vi "OAT Tachless Remove Control Point.vi"(10 "Pop Pos":cluster{i32, i32}, 11 "Tracks Ref":refnum<vi>) -> ()   [LabVIEW 2017, in "SoundVib_Tachless.lvlib"]
uses:
  <vilib>/addons/Sound and Vibration/Order Analysis/Tachless/SoundVib_Tachless.lvlib
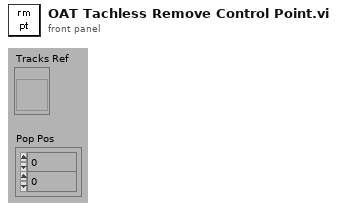
[diagram p1: front panel]
types:
  T1 = cluster{"Name":string, "Color":u32, "Style":u8, "Point Style":u8, "Name Visible":bool, "Allow Drag":bool, "Lock Style":u32, "Plot":u32, "Index":i32, "Position":cluster{"X":dbl, "Y":dbl}}[]
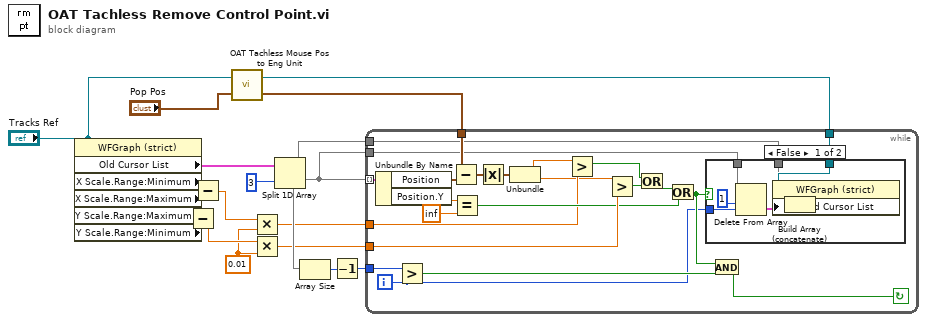
[diagram p0: block diagram]
diagram:
  w2 = 0.01 ("y")
  n1 = property on="Property Node" class="WFGraph (strict)"(reference="Tracks Ref") -> ("Old Cursor List"=w17:T1, "X Scale.Range:Minimum"=w11:dbl, "X Scale.Range:Maximum"=w12:dbl, "Y Scale.Range:Maximum"=w7:dbl, "Y Scale.Range:Minimum"=w6:dbl)  [unwired: 1 in, 2 out]
  n2 = Subtract(x=w7, y=w6) -> (x-y=w5:dbl)
  n3 = Subtract(x=w12, y=w11) -> (x-y=w3:dbl)
  n4 = call <vilib>:"OAT Tachless Mouse Pos to Eng Unit.vi"("Pop Pos"="Pop Pos", "Tracks ref"="Tracks Ref") -> ("Control Point"=w13:cluster{dbl, dbl})  [unwired: 1 in]
  n5 = Multiply(x=w3, y=w2) -> (x*y=w1:dbl)
  n6 = Multiply(x=w5, y=w2) -> (x*y=w4:dbl)
  n7 = Split 1D Array(array=w17, index=3 ("Array Index")) -> (first subarray=w9:T1, second subarray=w8:T1)
  n8 = Array Size(array=w8) -> (size(s)=w15:i32)
  n9 = Decrement(x=w15) -> (x-1=w14:i32)
  n10 = while {
    tunnel: w1 -> [w22]
    tunnel: w8 -> [w25]
    tunnel: w9 -> [w26]
    tunnel: "Tracks Ref" -> [w27]
    tunnel: w4 -> [w36]
    tunnel: w13 -> [w38]
    tunnel: w14 -> [w40]
    tunnel: w8 -> [w41] mode=indexing
    i -> [w24]
    stop <- w28 continue-if-true
    n11 = Unbundle By Name(w41) -> ("Position"=w39:cluster{"X":dbl, "Y":dbl}, "Position.Y"=w33:dbl)
    n12 = Greater?(x=w40, y=w24) -> (0:w29:bool)
    n13 = Subtract(x=w38, y=w39) -> (x-y=w34:cluster{dbl, dbl})
    n14 = Equal?(x=w33, y=inf) -> (x = y?=w31:bool)
    n15 = Absolute Value(x=w34) -> (abs(x)=w37:cluster{dbl, dbl})
    n16 = Unbundle(w37) -> (w23:dbl, w21:dbl)
    n17 = Greater?(x=w23, y=w22) -> (0:w19:bool)
    n18 = Greater?(x=w21, y=w36) -> (0:w35:bool)
    n19 = Or(x=w19, y=w35) -> (x .or. y?=w20:bool)
    n20 = Or(x=w20, y=w31) -> (x .or. y?=w30:bool)
    n21 = case shown="False" w30 {
      tunnel: w27 -> [w48 _]
      tunnel: w26 -> [w47 _]
      tunnel: w25 -> [w45 _]
      tunnel: w24 -> [w44 _]
      frame False {
        n22 = Delete From Array(array=w45, length=1 ("Index"), index=w44) -> (array with subset deleted=w46:T1)  [unwired: 1 out]
        n23 = Build Array (concatenate)(w47, w46) -> (w42:T1)
        n24 = property on="Property Node" class="WFGraph (strict)"(reference=w48, "Old Cursor List"=w42) -> ()  [unwired: 1 in, 2 out]
      }
      frame True {
      }
    }
    n25 = And(x=w30, y=w29) -> (x .and. y?=w28:bool)
  }
